vi "Write_param.vi"   [LabVIEW 2018]
uses:
  Init/AllPath.vi
  <vilib>/Utility/file.llb/Write Delimited Spreadsheet (string).vi
types:
  T1 = cluster{"Selected Index []":i32[], "Selected Items":string[], " 所有任务":string[], "任务布尔":bool[]}
  T2 = typedef "IMAQ Image.ctl" = refnum<image>
  T3 = cluster{"示波器":cluster{"Channel (0:Channel 1)":enum16{"Channel 1", "Channel 2", "Channel 3", "Channel 4"}, "电压范围":dbl, "触发电压":dbl, "时间范围":dbl, " 示波器VISA":refnum<visa-resource-name>, "时间范围 标签":u64, "电压范围 标签":u64, "触发电压 标签":u64, "输入阻抗/Ω":u64}, "光谱仪":cluster{"SpecDataReference":refnum<queue>, "grating center":dbl, "Exposure Time (s)":dbl, "是否进行详细设置":bool, " 开始通信检查":bool, "通信成功？":bool, "波长":dbl}, " 近场相机":cluster{"曝光时间/us":dbl, "模拟增益":i32, "控制套接字":i32, "IP 地址":string, " 采集套接字":i32, "  版本号":i32, "ImageData":T2, "  增益最大":i32, "  增益最小":i32, " 曝光最大":i32, " 曝光最小":i32, " 帧速":i32, " 同步切换":i32, "  曝光缩放":i32, "Camera Source":refnum<k21>, "近场X范围":dbl, "近场Y范围":dbl, "单个像元大小/um":dbl, "相机距离原点位置":dbl[], "是否测量发散角":bool, "光束类型":bool}, " 偏振仪":cluster{"电压范围":u64, "触发电压":u64, "时间范围":u64, "波长范围":enum16{"可见光 400-700nm", "近红外 700-1100nm"}, "可见光偏振测量仪VISA":refnum<visa-resource-name>, "近红外偏振测量仪VISA":refnum<visa-resource-name>}, " 功率计":cluster{"通道":enum16{"Channel 1", "Channel 2"}, "工作波长":u32, "单位":u64, "时间范围":u64, "IP地址":string, "端口":u32, "是否需要散射片":bool}, "能量计":cluster{"通道":enum16{"Channel 1", "Channel 2"}, "工作波长":u32, "单位":u64, "时间范围":u64, "IP地址":string, "端口":u32, "能量计量程":enum16{"200uJ", "20uJ", "2uJ", "200nJ"}}, "电机":cluster{"Channel (0:Channel 1)":enum16{"Channel 1", "Channel 2", "Channel 3", "Channel 4"}, "电压范围":u64, "触发电压":u64, "时间范围":u64}, " 远场相机":cluster{"曝光时间":i32, "模拟增益":i32, "控制套接字":i32, "IP 地址":string, " 采集套接字":i32, "  版本号":i32, "ImageData":T2, "  增益最大":i32, "  增益最小":i32, " 曝光最大":i32, " 曝光最小":i32, " 帧速":i32, " 同步切换":i32, "  曝光缩放":i32, "ImageData B":T2}}
  T4 = enum16{"Channel 1", "Channel 2", "Channel 3", "Channel 4"}
  T5 = cluster{"激光器型号":string, "X":dbl, "Y":dbl, "Z":dbl, "Rotate":dbl, "Pitching":dbl, "DivergeAngle":dbl}
  T6 = cluster{"能量/功率":path, " 示波器":path, " 光谱仪":path, "偏振":path, "近远场":cluster{" 近场图片":path, " 远场图片":path, "发散角数据":path}, "参数":path, " 基路径":path, "文件名信息":path}
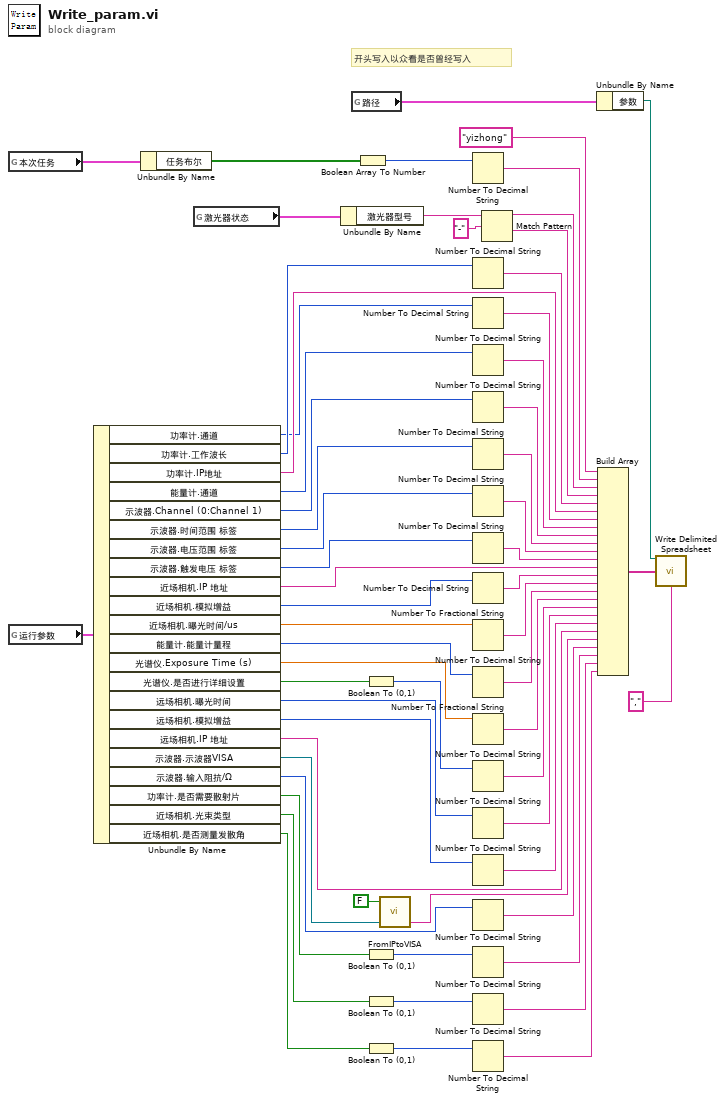
[diagram p0: block diagram]
diagram:
  # "开头写入以众看是否曾经写入"
  n1 = global read "参数.vi" "本次任务"() -> (w30:T1)
  n2 = global read "参数.vi" "运行参数"() -> (w61:T3)
  n3 = Unbundle By Name(w61) -> ("功率计.通道"=w32:enum16{"Channel 1", "Channel 2"}, "功率计.工作波长"=w33:u32, "功率计.IP地址"=w54:string, "能量计.通道"=w52:enum16{"Channel 1", "Channel 2"}, "示波器.Channel (0:Channel 1)"=w50:T4, "示波器.时间范围 标签"=w48:u64, "示波器.电压范围 标签"=w47:u64, "示波器.触发电压 标签"=w44:u64, "近场相机.IP 地址"=w42:string, "近场相机.模拟增益"=w41:i32, "近场相机.曝光时间/us"=w40:dbl, "能量计.能量计量程"=w26:enum16{"200uJ", "20uJ", "2uJ", "200nJ"}, "光谱仪.Exposure Time (s)"=w24:dbl, "光谱仪.是否进行详细设置"=w22:bool, "远场相机.曝光时间"=w19:i32, "远场相机.模拟增益"=w18:i32, "远场相机.IP 地址"=w15:string, "示波器.示波器VISA"=w13:refnum<visa-resource-name>, "示波器.输入阻抗/Ω"=w11:u64, "功率计.是否需要散射片"=w9:bool, "近场相机.光束类型"=w8:bool, "近场相机.是否测量发散角"=w7:bool)
  n4 = Unbundle By Name(w30) -> ("任务布尔"=w29:bool[])
  n5 = global read "参数.vi" "激光器状态"() -> (w60:T5)
  n6 = Unbundle By Name(w60) -> ("激光器型号"=w59:string)
  n7 = global read "AllPath.vi" "路径"() -> (w37:T6)
  n8 = Boolean Array To Number(Boolean array=w29) -> (number=w28:u32)
  n9 = Boolean To (0,1)(Boolean=w22) -> (0, 1=w21:i16)
  n10 = Boolean To (0,1)(Boolean=w9) -> (0, 1=w3:i16)
  n11 = Boolean To (0,1)(Boolean=w8) -> (0, 1=w2:i16)
  n12 = Boolean To (0,1)(Boolean=w7) -> (0, 1=w1:i16)
  n13 = call "FromIPtoVISA.vi"("VISA in"=w13, "IP to VISA?"=FALSE) -> ("IP  out"=w12:string)  [unwired: 2 in, 1 out]
  n14 = Number To Decimal String(number=w28) -> (decimal integer string=w27:string)  [unwired: 1 in]
  n15 = Number To Decimal String(number=w33) -> (decimal integer string=w55:string)  [unwired: 1 in]
  n16 = Number To Decimal String(number=w32) -> (decimal integer string=w53:string)  [unwired: 1 in]
  n17 = Number To Decimal String(number=w52) -> (decimal integer string=w51:string)  [unwired: 1 in]
  n18 = Number To Decimal String(number=w50) -> (decimal integer string=w49:string)  [unwired: 1 in]
  n19 = Number To Decimal String(number=w48) -> (decimal integer string=w46:string)  [unwired: 1 in]
  n20 = Number To Decimal String(number=w47) -> (decimal integer string=w45:string)  [unwired: 1 in]
  n21 = Number To Decimal String(number=w44) -> (decimal integer string=w43:string)  [unwired: 1 in]
  n22 = Number To Decimal String(number=w41) -> (decimal integer string=w39:string)  [unwired: 1 in]
  n23 = Number To Fractional String(number=w40) -> (F-format string=w38:string)  [unwired: 3 in]
  n24 = Number To Decimal String(number=w26) -> (decimal integer string=w25:string)  [unwired: 1 in]
  n25 = Number To Fractional String(number=w24) -> (F-format string=w23:string)  [unwired: 3 in]
  n26 = Number To Decimal String(number=w21) -> (decimal integer string=w20:string)  [unwired: 1 in]
  n27 = Number To Decimal String(number=w19) -> (decimal integer string=w17:string)  [unwired: 1 in]
  n28 = Number To Decimal String(number=w18) -> (decimal integer string=w16:string)  [unwired: 1 in]
  n29 = Number To Decimal String(number=w11) -> (decimal integer string=w10:string)  [unwired: 1 in]
  n30 = Number To Decimal String(number=w3) -> (decimal integer string=w6:string)  [unwired: 1 in]
  n31 = Number To Decimal String(number=w2) -> (decimal integer string=w5:string)  [unwired: 1 in]
  n32 = Number To Decimal String(number=w1) -> (decimal integer string=w4:string)  [unwired: 1 in]
  n33 = Match Pattern(string=w59, regular expression="-" ("正则表达式")) -> (before substring=w57:string, after substring=w56:string)  [unwired: 1 in, 2 out]
  n34 = Unbundle By Name(w37) -> ("参数"=w36:path)
  n35 = Build Array("yizhong" ("元素"), w27, w57, w56, w55, w54, w53, w51, w49, w46, w45, w43, w42, w39, w38, w25, w23, w20, w17, w16, w15, w12, w10, w6, w5, w4) -> (w35:string[])
  n36 = call-poly <vilib>:"Write Delimited Spreadsheet.vi"("file path (dialog if empty)"=w36, "1D data"=w35, "delimiter (\\t)"="," ("delimiter (\\t)")) -> ()  [unwired: 11 in, 2 out]
